vi "Close.vi"(8 "error in":errorcluster, 11 "SimpleCsvDataLogger in":refnum<class "SimpleCsvDataLogger.lvclass">) -> (0 "error out":errorcluster, 3 "SimpleCsvDataLogger out":refnum<class "SimpleCsvDataLogger.lvclass">)   [LabVIEW 2024, in "SimpleCsvDataLogger.lvclass"]
uses:
  SimpleCsvDataLogger.lvclass
  SimpleCsvDataLogger.lvclass/SimpleCsvDataLogger.ctl
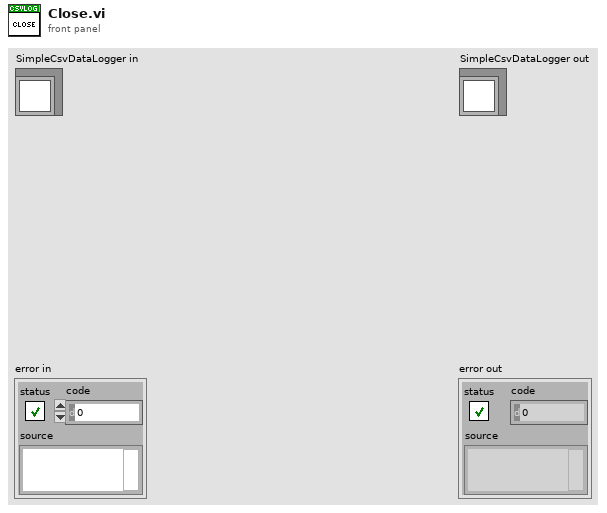
[diagram p1: front panel]
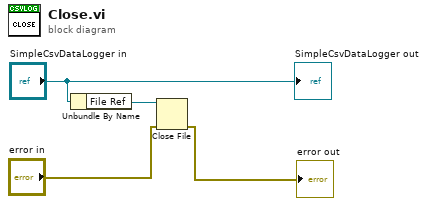
[diagram p0: block diagram]
diagram:
  n1 = Unbundle By Name("SimpleCsvDataLogger in") -> ("File Ref"=w3:refnum<file>)
  n2 = Close File(refnum=w3, error in="error in") -> (error out=→"error out":errorcluster)  [unwired: 1 out]
  "SimpleCsvDataLogger out" <- "SimpleCsvDataLogger in"
